vi "WSVCAP SHL Host TL I2C Write - Multiple Device - Unique Data.vi"(0 "C1 Data":u8[](array[numeric]) format="%.0x", 1 "Sub Address":u8=20 format="%.0x", 3 "FPGA":T1, 11 "error in":errorcluster, 12 "Log (T)":bool=TRUE, 13 "DUT Mask Array (All)":bool[](array[boolean])=[TRUE, TRUE, TRUE, TRUE, TRUE, TRUE, TRUE, TRUE, TRUE, TRUE, TRUE, TRUE, TRUE, TRUE, TRUE, TRUE, TRUE, TRUE, TRUE, TRUE, TRUE, TRUE, TRUE, TRUE, TRUE, TRUE, TRUE, TRUE, TRUE, TRUE, TRUE, TRUE, TRUE, TRUE, TRUE, TRUE, TRUE, TRUE, TRUE, TRUE, TRUE, TRUE, TRUE, TRUE, TRUE, TRUE, TRUE, TRUE, TRUE, TRUE, TRUE, TRUE, TRUE, TRUE, TRUE, TRUE, TRUE, TRUE, TRUE, TRUE, TRUE, TRUE, TRUE, TRUE], 14 "DUT Mask Mode (All)":T2=enum."All") -> (15 "error out":errorcluster)   [LabVIEW 2017]
uses:
  Type Defs/WSVCAP SHL I2C DUT Mask Mode Enum.ctl
  Type Defs/WSVCAP SHL FPGA Enum.ctl
panel:
  out "Socket Mask [U64]":u64 format="%016x"
  out "C1 Data Out":u8[](array[numeric]) format="%.0x"
  # "DUT 01"
  # "DUT 02"
  # "DUT 03"
  # "DUT 04"
  # "DUT 05"
  # "DUT 06"
  # "DUT 07"
  # "DUT 08"
  # "DUT 09"
  # "DUT 10"
  # "DUT 11"
  # "DUT 12"
  # "DUT 13"
  # "DUT 14"
  # "DUT 15"
  # "DUT 16"
  # "DUT 17"
  # "DUT 18"
  # "DUT 19"
  # "DUT 20"
  # "DUT 21"
  # "DUT 22"
  # "DUT 23"
  # "DUT 24"
  # "C"
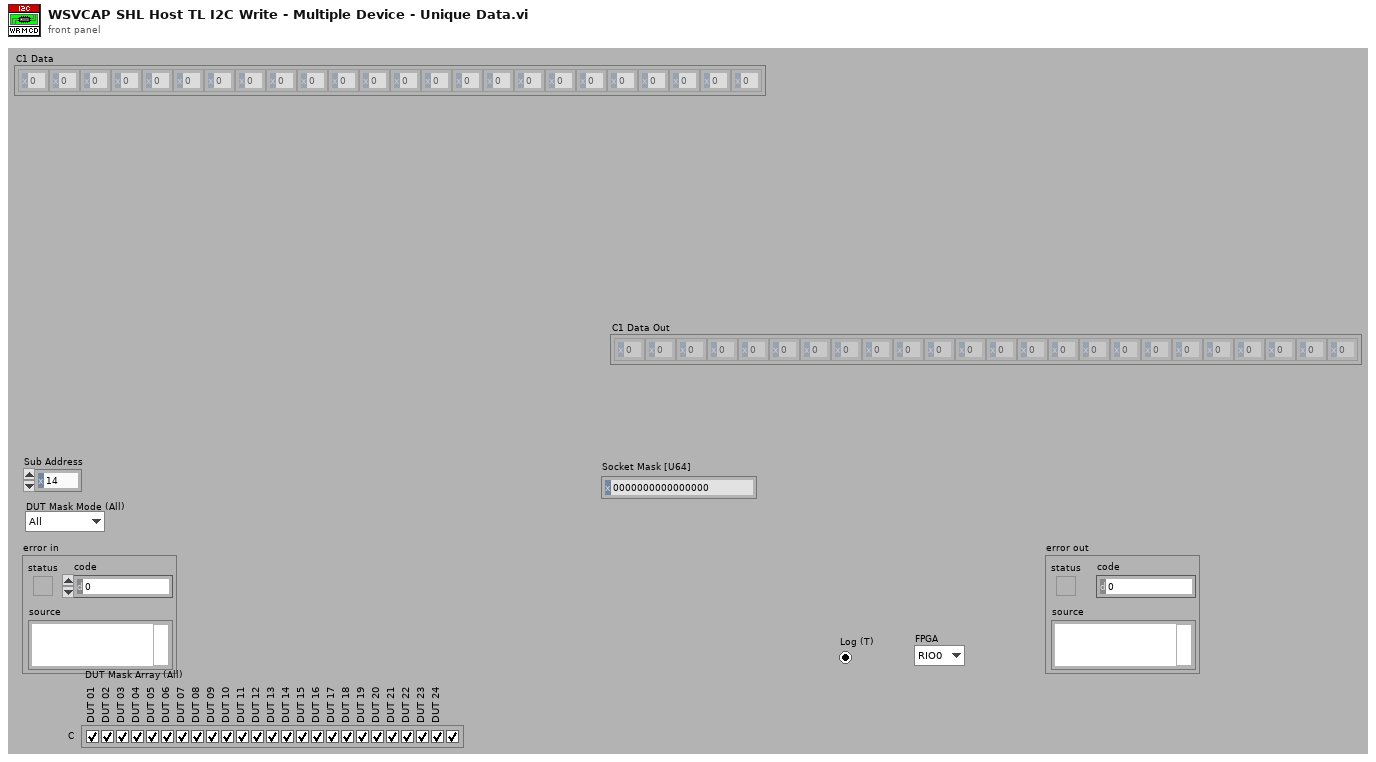
[diagram p1: front panel]
types:
  T1 = typedef "WSVCAP SHL FPGA Enum.ctl" = enum16{"RIO0", "RIO1"}
  T2 = typedef "WSVCAP SHL I2C DUT Mask Mode Enum.ctl" = enum16{"Custom", "All"}
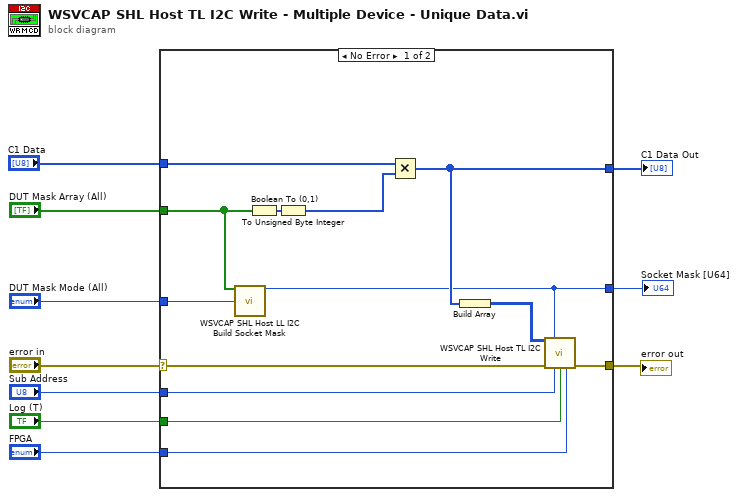
[diagram p0: block diagram]
diagram:
  n1 = case shown="No Error" "error in" {
    selector: "error in" -> [w19 w24]
    tunnel: [w23 w24] -> w10
    tunnel: "Sub Address" -> [w17 _]
    tunnel: [w20 _] -> w7
    tunnel: [w13 _] -> w6
    tunnel: "DUT Mask Array (All)" -> [w11 _]
    tunnel: "Log (T)" -> [w18 _]
    tunnel: "DUT Mask Mode (All)" -> [w16 _]
    tunnel: "C1 Data" -> [w15 _]
    tunnel: "FPGA" -> [w14 _]
    frame No Error {
      n2 = call "WSVCAP SHL Host LL I2C Build Socket Mask.vi"("DUT Mask Array (All)"=w11, "DUT Mask Mode (Custom)"=w16) -> ("Socket Mask Set [U64]"=w13:u64)  [unwired: 13 in]
      n3 = Boolean To (0,1)(Boolean=w11) -> (0, 1=w21:i16[])
      n4 = To Unsigned Byte Integer(number=w21) -> (unsigned 8bit integer=w12:u8[])
      n5 = Multiply(x=w15, y=w12) -> (x*y=w20:u8[])
      n6 = Build Array(w20) -> (w22:u8[][])
      n7 = call "WSVCAP SHL Host TL I2C Write.vi"("C Data Out"=w22, "Socket Mask [U64]"=w13, "error in"=w19, "Sub Address"=w17, "Log (T)"=w18, "FPGA"=w14) -> ("error out"=w23:errorcluster)  [unwired: 9 in]
    }
    frame Error {
    }
  }
  "error out" <- w10
  "C1 Data Out" <- w7
  "Socket Mask [U64]" <- w6
